vi "ex4-2.vi"() -> ()   [LabVIEW 2009]
uses:
  <vilib>/NXT/Dual Mode Library/Motors/MotorOn.vi
  <vilib>/NXT/Dual Mode Library/Sensors/Touch_Pressed.vi
  <vilib>/NXT/Dual Mode Library/Sensors/Sonar_cm.vi
panel:
  out "距離(cm)":dbl
  out "是否壓下?":bool
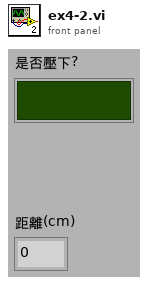
[diagram p1: front panel]
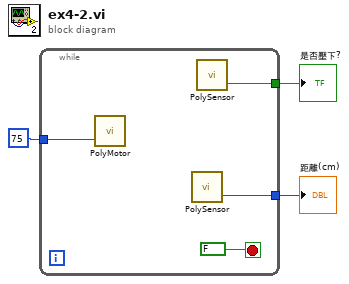
[diagram p0: block diagram]
diagram:
  n1 = while {
    tunnel: i8 75 ("Power (75)") -> [w6]
    tunnel: [w5] -> w2
    tunnel: [w4] -> w1
    stop <- FALSE stop-if-true
    n2 = call-poly <vilib>:"PolyMotor.vi"("Power (75)"=w6) -> ()  [unwired: 3 in, 1 out]
    n3 = call-poly <vilib>:"PolySensor.vi"() -> ("Distance (cm)"=w4:i16)  [unwired: 3 in, 1 out]
    n4 = call-poly <vilib>:"PolySensor.vi"() -> ("Yes / No"=w5:bool)  [unwired: 3 in, 1 out]
  }
  "是否壓下?" <- w2
  "距離(cm)" <- w1
